vi "excercise1.vi"() -> ()   [LabVIEW 2013]
doc: "Use this template to build a producer/consumer design pattern with events to produce queue items. Use this design pattern instead of the User Interface Event Handler pattern for user interfaces when you want to execute code asynchronously in response to an event without slowing the user interface responsiveness."
uses:
  controls/clsData.ctl
panel:
  out "plotNames":string[](array[string])
  out "graph":dbl[][](graph)
  in  "Size":u32=50 min=1 step=1
  in  "b":dbl
  in  "m":dbl
  in  "Clear Graph":bool
  in  "Add Plot":bool
  in  "stop":bool
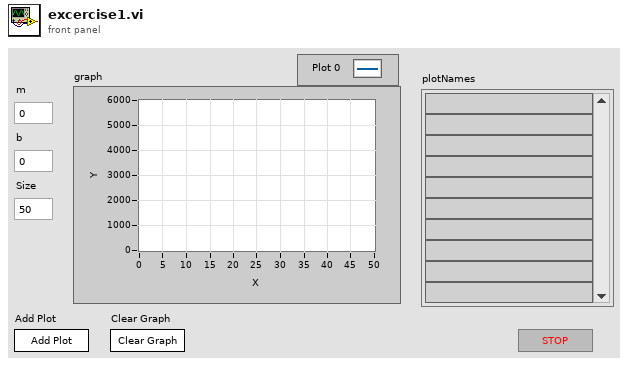
[diagram p1: front panel]
types:
  T1 = typedef "clsData.ctl" = cluster{"Cmd":string, "m":dbl, "b":dbl, "Size":u32}
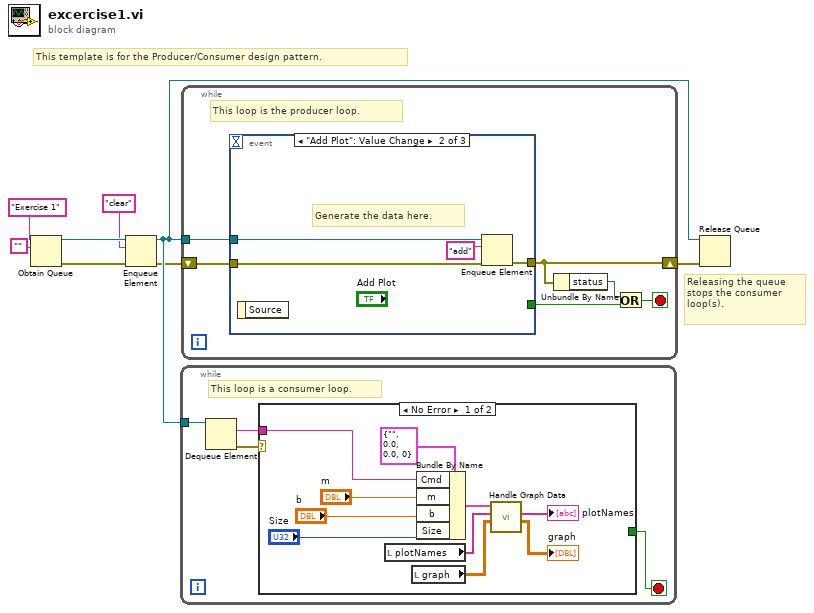
[diagram p0: block diagram]
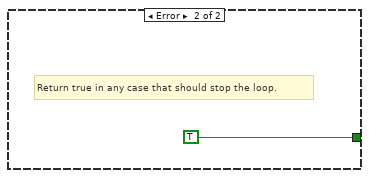
[diagram p2: hidden frame]
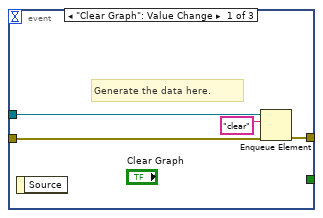
[diagram p3: hidden frame]
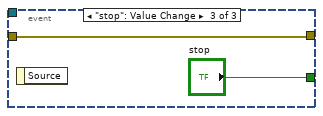
[diagram p4: hidden frame]
diagram:
  # "Releasing the queue stops the consumer loop(s)."
  # "This template is for the Producer/Consumer design pattern."
  n1 = Obtain Queue(name (unnamed)="Exercise 1", element data type="" ("data (can be any type)")) -> (queue out=w5:refnum<queue>, error out=w3:errorcluster)  [unwired: 3 in, 1 out]
  n2 = Enqueue Element(queue=w5, element="clear", error in (no error)=w3) -> (queue out=w4:refnum<queue>, error out=w2:errorcluster)  [unwired: 1 in, 1 out]
  n3 = while {
    tunnel: w4 -> [w12]
    stop <- w9 stop-if-true
    # "This loop is a consumer loop."
    n4 = Dequeue Element(queue=w12) -> (element=w10:string, error out=w11:errorcluster)  [unwired: 2 in, 2 out]
    n5 = case shown="No Error" w11 {
      tunnel: w10 -> [w18 _]
      tunnel: [_ TRUE] -> w9
      frame No Error {
        n6 = local read "plotNames"() -> (w16:string[])
        n7 = local read "graph"() -> (w15:dbl[][])
        n8 = Bundle By Name(cluster=T1 {"Cmd"="", "m"=0.0, "b"=0.0, "Size"=0} ("clsData"), "Cmd"=w18, "m"="m", "b"="b", "Size"="Size") -> (w17:T1)
        n9 = call "Handle Graph Data.vi"("graph in"=w15, "plotNames in"=w16, "clsData"=w17) -> ("graph out"=→"graph":dbl[][], "plotNames out"=→"plotNames":string[])  [unwired: 6 in, 1 out]
      }
      frame Error {
        # "Return true in any case that should stop the loop."
      }
    }
  }
  n10 = while {
    shift-right: [w25] -> w8
    shift-left: w2 -> [w28]
    tunnel: w4 -> [w29]
    stop <- w26 stop-if-true
    # "This loop is the producer loop."
    n11 = event shown="[1] \"Add Plot\": Value Change" {
      selector: _ -> [_ _ _]
      dyn-events: _ -> [_ _ _]
      timeout: _ -> [_ _ _]
      tunnel: w29 -> [w33 w37 _]
      tunnel: w28 -> [w32 w36 w38]
      tunnel: [w31 w35 w38] -> w25
      tunnel: [_ _ "stop"] -> w27
      event "Clear Graph": Value Change {
        # "Generate the data here."
        n12 = event-data() -> ()  [unwired: 1 in, 1 out]
        n13 = Enqueue Element(queue=w33, element="clear", error in (no error)=w32) -> (error out=w31:errorcluster)  [unwired: 1 in, 2 out]
      }
      event "Add Plot": Value Change {
        # "Generate the data here."
        n14 = event-data() -> ()  [unwired: 1 in, 1 out]
        n15 = Enqueue Element(queue=w37, element="add", error in (no error)=w36) -> (error out=w35:errorcluster)  [unwired: 1 in, 2 out]
      }
      event "stop": Value Change {
        n16 = event-data() -> ()  [unwired: 1 in, 1 out]
      }
    }
    n17 = Unbundle By Name(w25) -> ("status"=w24:bool)
    n18 = Or(x=w24, y=w27) -> (x .or. y?=w26:bool)
  }
  n19 = Release Queue(queue=w4, error in (no error)=w8) -> ()  [unwired: 1 in, 3 out]
